vi "Status.vi"(8 "error in (no error)":errorcluster, 11 "4-20mA Out Settings In":T1) -> (0 "error out":errorcluster, 1 "Connection Error":bool, 2 "Pump On?":enum16{"Off", "On", "Not Initialized"}(ring), 3 "4-20mA Out Settings Out":T1)   [LabVIEW 2018, in "Flow Regulator Library.lvlib"]
uses:
  Pressure Reg Module/Flow Regulator Library.lvlib
  Pressure Reg Module/Pressure Regulator Device Settings.ctl
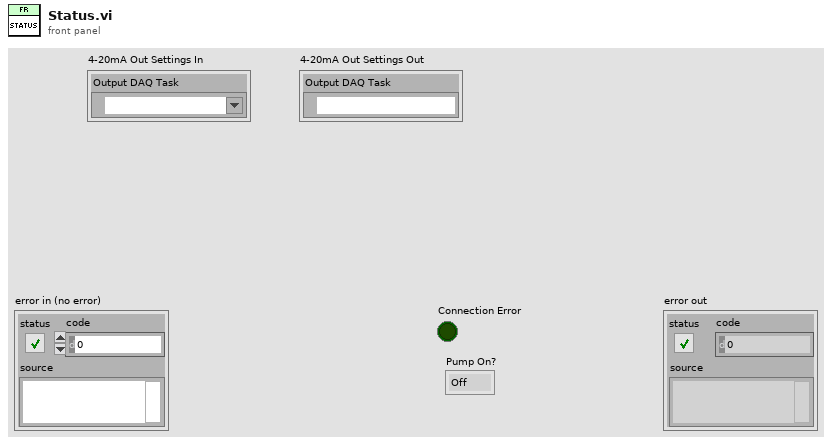
[diagram p1: front panel]
types:
  T1 = typedef "Flow Regulator Library.lvlib/Pressure Regulator Device Settings.ctl" = cluster{"Output DAQ Task":refnum<k21>}
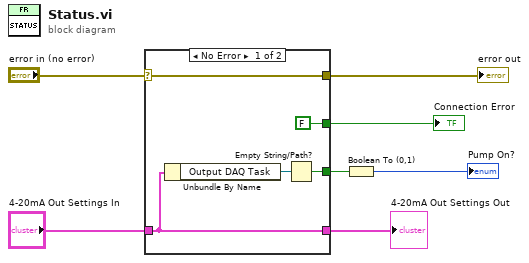
[diagram p0: block diagram]
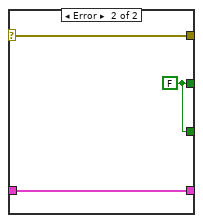
[diagram p2: hidden frame]
diagram:
  n1 = case shown="No Error" "error in (no error)" {
    selector: "error in (no error)" -> [w8 w15]
    tunnel: [w8 w15] -> w6
    tunnel: "4-20mA Out Settings In" -> [w10 w14]
    tunnel: [w10 w14] -> w4
    tunnel: [FALSE w13] -> w3
    tunnel: [w9 w13] -> w1
    frame No Error {
      n2 = Unbundle By Name(w10) -> ("Output DAQ Task"=w12:refnum<k21>)
      n3 = Empty String/Path?(string/path=w12) -> (empty?=w9:bool)
    }
    frame Error {
      w13 = FALSE
    }
  }
  "error out" <- w6
  "Connection Error" <- w3
  "4-20mA Out Settings Out" <- w4
  n4 = Boolean To (0,1)(Boolean=w1) -> (0, 1=→"Pump On?":i16)
